vi "All Tubes ON - OFF.vi"(6 "Tubes ON/OFF":bool, 7 "Numeric":i32=65) -> ()   [LabVIEW 2020]
uses:
  <vilib>/DAQmx/write.llb/DAQmx Write (Digital U8 1Chan 1Samp).vi
  <vilib>/DAQmx/create/channels.llb/DAQmx Create Channel (DO-Digital Output).vi
  <vilib>/DAQmx/miscellaneous.llb/DAQmx Fill In Error Info.vi
panel:
  out "Status(U8) 2":u8
  in  "lines 2":tag="Dev2/port0/line0:7"
  out "Status(U8)":u8
  in  "lines":tag="Dev2/port0/line0:7"
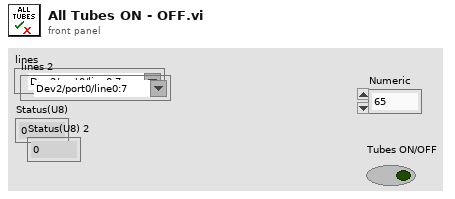
[diagram p1: front panel]
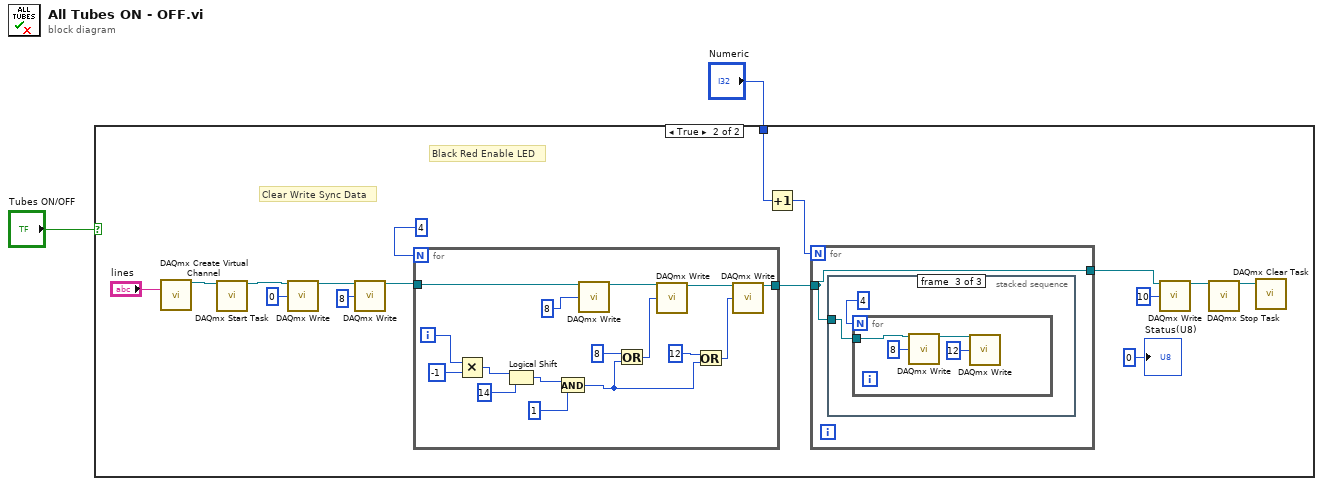
[diagram p0: block diagram]
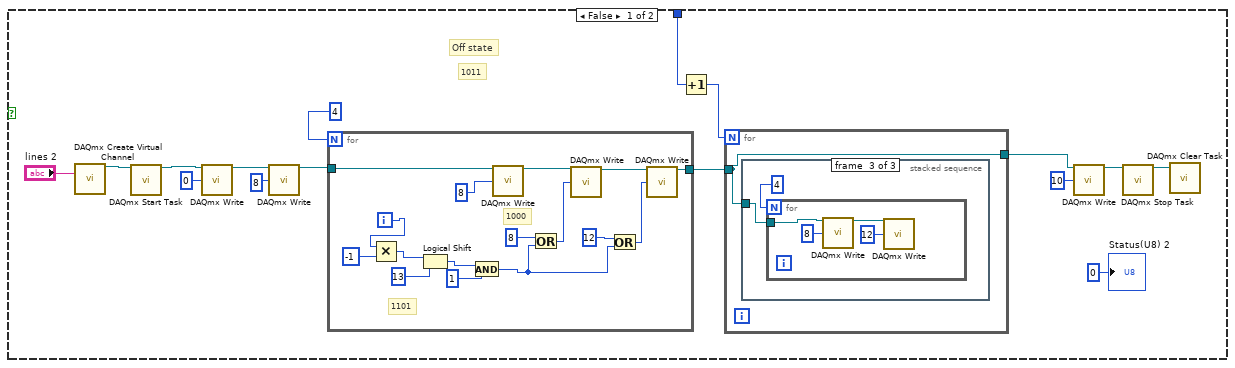
[diagram p2: hidden frame]
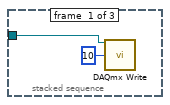
[diagram p3: hidden frame]
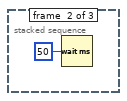
[diagram p4: hidden frame]
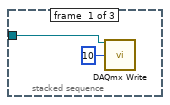
[diagram p5: hidden frame]
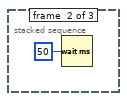
[diagram p6: hidden frame]
diagram:
  n1 = case shown="True" "Tubes ON/OFF" {
    tunnel: "Numeric" -> [w3 w45]
    frame False {
      # "Off state"
      # "1011"
      n2 = call-poly <vilib>:"DAQmx Create Virtual Channel.vi"("lines"="lines 2") -> ("task out"=w18:refnum<k21>)  [unwired: 13 in, 1 out]
      n3 = call <vilib>:"DAQmx Start Task.vi"("task/channels in"=w18) -> ("task out"=w10:refnum<k21>)  [unwired: 13 in, 1 out]
      n4 = call-poly <vilib>:"DAQmx Write.vi"("task/channels in"=w10, "data"=u8 0) -> ("task out"=w9:refnum<k21>)  [unwired: 11 in, 2 out]
      n5 = call-poly <vilib>:"DAQmx Write.vi"("task/channels in"=w9, "data"=u8 8) -> ("task out"=w14:refnum<k21>)  [unwired: 11 in, 2 out]
      n6 = for {
        N: 4 -> [_]
        tunnel: w14 -> [w33]
        tunnel: [w30] -> w7
        i -> [w42]
        # "1000"
        # "1101"
        n7 = Multiply(x=w42, y=-1) -> (x*y=w40:i32)
        n8 = Logical Shift(y=w40, x=u8 13) -> (x << y=w44:u8)
        n9 = And(x=w44, y=u32 1) -> (x .and. y?=w36:u32)
        n10 = call-poly <vilib>:"DAQmx Write.vi"("task/channels in"=w33, "data"=u32 8 ("x")) -> ("task out"=w32:refnum<k21>)  [unwired: 11 in, 2 out]
        n11 = Or(x=u32 8, y=w36) -> (x .or. y?=w37:u32)
        n12 = call-poly <vilib>:"DAQmx Write.vi"("task/channels in"=w32, "data"=w37) -> ("task out"=w31:refnum<k21>)  [unwired: 11 in, 2 out]
        n13 = Or(x=u32 12, y=w36) -> (x .or. y?=w34:u32)
        n14 = call-poly <vilib>:"DAQmx Write.vi"("task/channels in"=w31, "data"=w34) -> ("task out"=w30:refnum<k21>)  [unwired: 11 in, 2 out]
      }
      n15 = Increment(x=w3) -> (x+1=w4:i32)
      n16 = for {
        N: w4 -> [_]
        tunnel: w7 -> [w19]
        tunnel: [w19] -> w6
        n17 = stacked-sequence {
          tunnel: w19 -> [w20 _ w23]
          frame #0 {
            n18 = call-poly <vilib>:"DAQmx Write.vi"("task/channels in"=w20, "data"=u8 10) -> ()  [unwired: 11 in, 3 out]
          }
          frame #1 {
            n19 = Wait (ms)(milliseconds to wait=u32 50) -> ()  [unwired: 1 out]
          }
          frame #2 {
            n20 = for {
              N: 4 -> [_]
              tunnel: w23 -> [w26]
              n21 = call-poly <vilib>:"DAQmx Write.vi"("task/channels in"=w26, "data"=u8 8) -> ("task out"=w25:refnum<k21>)  [unwired: 11 in, 2 out]
              n22 = call-poly <vilib>:"DAQmx Write.vi"("task/channels in"=w25, "data"=u8 12) -> ()  [unwired: 11 in, 3 out]
            }
          }
        }
      }
      n23 = call-poly <vilib>:"DAQmx Write.vi"("task/channels in"=w6, "data"=u8 10) -> ("task out"=w13:refnum<k21>)  [unwired: 11 in, 2 out]
      n24 = call <vilib>:"DAQmx Stop Task.vi"("task/channels in"=w13) -> ("task out"=w17:refnum<k21>)  [unwired: 13 in, 1 out]
      n25 = call <vilib>:"DAQmx Clear Task.vi"("task in"=w17) -> ()  [unwired: 14 in, 1 out]
      "Status(U8) 2" <- u8 0
    }
    frame True {
      # "Black Red Enable LED"
      # "Clear Write Sync Data"
      n26 = call-poly <vilib>:"DAQmx Create Virtual Channel.vi"("lines"="lines") -> ("task out"=w60:refnum<k21>)  [unwired: 13 in, 1 out]
      n27 = call <vilib>:"DAQmx Start Task.vi"("task/channels in"=w60) -> ("task out"=w52:refnum<k21>)  [unwired: 13 in, 1 out]
      n28 = call-poly <vilib>:"DAQmx Write.vi"("task/channels in"=w52, "data"=u8 0) -> ("task out"=w51:refnum<k21>)  [unwired: 11 in, 2 out]
      n29 = call-poly <vilib>:"DAQmx Write.vi"("task/channels in"=w51, "data"=u8 8) -> ("task out"=w56:refnum<k21>)  [unwired: 11 in, 2 out]
      n30 = for {
        N: 4 -> [_]
        tunnel: w56 -> [w75]
        tunnel: [w72] -> w49
        i -> [w84]
        n31 = Multiply(x=w84, y=-1) -> (x*y=w82:i32)
        n32 = Logical Shift(y=w82, x=u8 14) -> (x << y=w86:u8)
        n33 = And(x=w86, y=u32 1) -> (x .and. y?=w78:u32)
        n34 = call-poly <vilib>:"DAQmx Write.vi"("task/channels in"=w75, "data"=u32 8 ("x")) -> ("task out"=w74:refnum<k21>)  [unwired: 11 in, 2 out]
        n35 = Or(x=u32 8, y=w78) -> (x .or. y?=w79:u32)
        n36 = call-poly <vilib>:"DAQmx Write.vi"("task/channels in"=w74, "data"=w79) -> ("task out"=w73:refnum<k21>)  [unwired: 11 in, 2 out]
        n37 = Or(x=u32 12, y=w78) -> (x .or. y?=w76:u32)
        n38 = call-poly <vilib>:"DAQmx Write.vi"("task/channels in"=w73, "data"=w76) -> ("task out"=w72:refnum<k21>)  [unwired: 11 in, 2 out]
      }
      n39 = Increment(x=w45) -> (x+1=w46:i32)
      n40 = for {
        N: w46 -> [_]
        tunnel: w49 -> [w61]
        tunnel: [w61] -> w48
        n41 = stacked-sequence {
          tunnel: w61 -> [w62 _ w65]
          frame #0 {
            n42 = call-poly <vilib>:"DAQmx Write.vi"("task/channels in"=w62, "data"=u8 10) -> ()  [unwired: 11 in, 3 out]
          }
          frame #1 {
            n43 = Wait (ms)(milliseconds to wait=u32 50) -> ()  [unwired: 1 out]
          }
          frame #2 {
            n44 = for {
              N: 4 -> [_]
              tunnel: w65 -> [w68]
              n45 = call-poly <vilib>:"DAQmx Write.vi"("task/channels in"=w68, "data"=u8 8) -> ("task out"=w67:refnum<k21>)  [unwired: 11 in, 2 out]
              n46 = call-poly <vilib>:"DAQmx Write.vi"("task/channels in"=w67, "data"=u8 12) -> ()  [unwired: 11 in, 3 out]
            }
          }
        }
      }
      n47 = call-poly <vilib>:"DAQmx Write.vi"("task/channels in"=w48, "data"=u8 10) -> ("task out"=w55:refnum<k21>)  [unwired: 11 in, 2 out]
      n48 = call <vilib>:"DAQmx Stop Task.vi"("task/channels in"=w55) -> ("task out"=w59:refnum<k21>)  [unwired: 13 in, 1 out]
      n49 = call <vilib>:"DAQmx Clear Task.vi"("task in"=w59) -> ()  [unwired: 14 in, 1 out]
      "Status(U8)" <- u8 0
    }
  }
